vi "Set Generic Property.vi"   [LabVIEW 2020, in "SLSC.lvlib"]
doc: "Sets the value of the specified device property for one or more resources. This is flexible for devices, NVMEM, physical channels, and so on, but requires that you know the exact string of the resource."
uses:
  <vilib>/SLSC/SLSC.lvlib
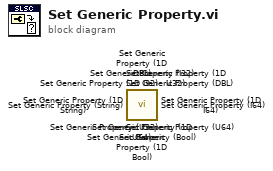
[diagram p0: block diagram]
diagram:
  n1 = call <vilib>:"Set Generic Property (1D U64).vi"() -> ()  [unwired: 14 in, 2 out]
  n2 = call <vilib>:"Set Generic Property (1D U32).vi"() -> ()  [unwired: 14 in, 2 out]
  n3 = call <vilib>:"Set Generic Property (1D String).vi"() -> ()  [unwired: 14 in, 2 out]
  n4 = call <vilib>:"Set Generic Property (1D I64).vi"() -> ()  [unwired: 14 in, 2 out]
  n5 = call <vilib>:"Set Generic Property (1D I32).vi"() -> ()  [unwired: 14 in, 2 out]
  n6 = call <vilib>:"Set Generic Property (1D DBL).vi"() -> ()  [unwired: 14 in, 2 out]
  n7 = call <vilib>:"Set Generic Property (1D Bool).vi"() -> ()  [unwired: 14 in, 2 out]
  n8 = call <vilib>:"Set Generic Property (U64).vi"() -> ()  [unwired: 14 in, 2 out]
  n9 = call <vilib>:"Set Generic Property (U32).vi"() -> ()  [unwired: 14 in, 2 out]
  n10 = call <vilib>:"Set Generic Property (String).vi"() -> ()  [unwired: 14 in, 2 out]
  n11 = call <vilib>:"Set Generic Property (I64).vi"() -> ()  [unwired: 14 in, 2 out]
  n12 = call <vilib>:"Set Generic Property (I32).vi"() -> ()  [unwired: 14 in, 2 out]
  n13 = call <vilib>:"Set Generic Property (DBL).vi"() -> ()  [unwired: 14 in, 2 out]
  n14 = call <vilib>:"Set Generic Property (Bool).vi"() -> ()  [unwired: 14 in, 2 out]
